vi "LibXML_CreateNewNode.vi"(8 "error in":errorcluster, 10 "name":string, 11 "doc":u32) -> (0 "error out":errorcluster, 2 "nodePtr out":u32, 3 "doc out":u32)   [LabVIEW 2019, in "Tools.lvlib" / "LibXML.lvlib"]
doc: "Create a new node in doc (U32) with specified name."
uses:
  LibXML.lvlib
  dll/libxml2.dll
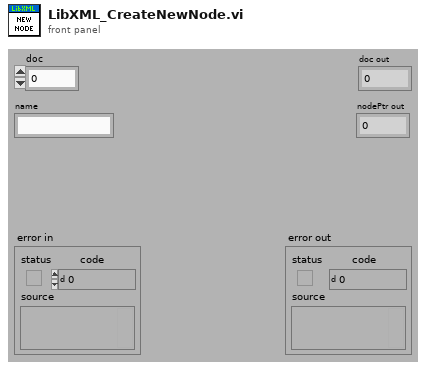
[diagram p1: front panel]
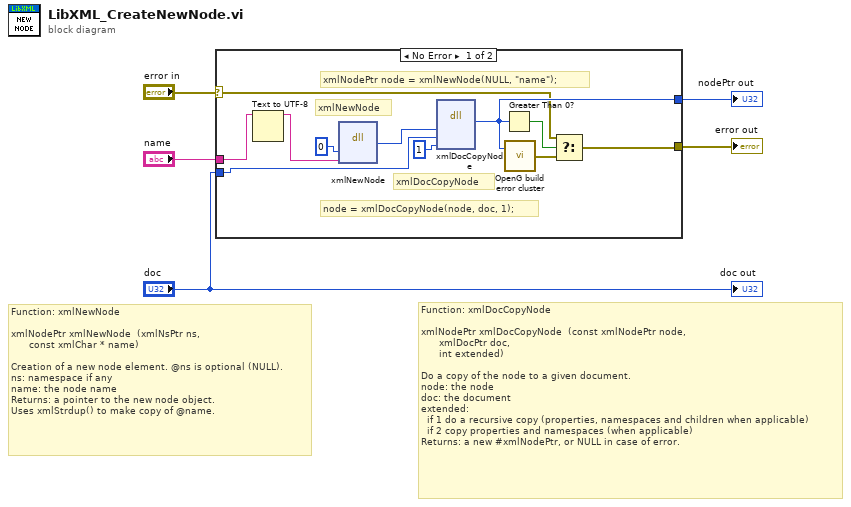
[diagram p0: block diagram]
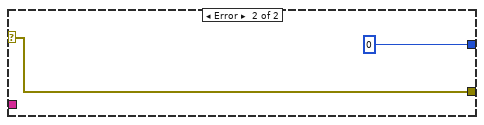
[diagram p2: hidden frame]
diagram:
  # "Function: xmlNewNode\n\nxmlNodePtr\txmlNewNode\t\t(xmlNsPtr ns, \n\t\t\t\t\t const xmlChar * name)\n\nCreation of a new node element. @ns is optional (NULL).\nns:\tnamespace if any\nname:\tthe node name\nReturns:\ta pointer to the new node object.\nUses xmlStrdup() to make copy of @name."
  # "Function: xmlDocCopyNode\n\nxmlNodePtr\txmlDocCopyNode\t\t(const xmlNodePtr node, \n\t\t\t\t\t xmlDocPtr doc, \n\t\t\t\t\t int extended)\n\nDo a copy of the node to a given document.\nnode:\tthe node\ndoc:\tthe document\nextended:\n \tif 1 do a recursive copy (properties, namespaces and children when applicable)\n  if 2 copy properties and namespaces (when applicable)\nReturns:\ta new #xmlNodePtr, or NULL in case of error."
  n1 = case shown="No Error" "error in" {
    selector: "error in" -> [w8 w18]
    tunnel: [w12 w18] -> w5
    tunnel: "doc" -> [w10 _]
    tunnel: [w9 u32 0 ("return type")] -> w2
    tunnel: "name" -> [w7 _]
    frame No Error {
      # "xmlDocCopyNode"
      # "xmlNewNode"
      # "node = xmlDocCopyNode(node, doc, 1);"
      # "xmlNodePtr node = xmlNewNode(NULL, \"name\");"
      n2 = Text to UTF-8(11:w7) -> (3:w6:string)  [unwired: 2 in, 1 out]
      n3 = dll-call lib="C:/Projects/_Prywatne/MyCIT/Framework/Tools/XML/LibXML/dll/libxml2.dll" fn="xmlNewNode"("NS"=u32 0, "name"=w6) -> ("return type"=w15:u32)  [unwired: 5 in, 2 out]
      n4 = dll-call lib="C:/Projects/_Prywatne/MyCIT/Framework/Tools/XML/LibXML/dll/libxml2.dll" fn="xmlDocCopyNode"("node"=w15, "doc"=w10, "style"=1) -> ("return type"=w9:u32)  [unwired: 6 in, 2 out]
      n5 = Greater Than 0?(x=w9) -> (x > 0?=w11:bool)
      n6 = call "OpenG build error cluster.vi"("code"=w9) -> ("error out"=w13:errorcluster)  [unwired: 1 in]
      n7 = Select(t=w8, s=w11, f=w13) -> (s? t:f=w12:errorcluster)
    }
    frame Error {
    }
  }
  "error out" <- w5
  "nodePtr out" <- w2
  "doc out" <- "doc"
